vi "rqp_Show FP.vi"(4 "Show in Debugger?":bool=TRUE, 6 "Message Priority":T1=enum."Normal", 7 "Caller in":refnum<class "Worker.lvclass">, 8 "error in":errorcluster, 9 "Data in":T2, 11 "Settings in":refnum<class "Settings.lvclass">) -> (0 "error out":errorcluster, 3 "dup Settings out":refnum<class "Settings.lvclass">, 5 "dup Caller out":refnum<class "Worker.lvclass">)   [LabVIEW 2017, in "Settings.lvclass"]
doc: "This VI sends a <b>Public API Request</b> message to an MHL case of the Worker that owns this VI.\n---\nShow the Front Panel of the Settings Worker's Main VI."
uses:
  Settings.lvclass
  C:/Program Files (x86)/National Instruments/LabVIEW 2017/vi.lib/addons/_Workers/Library/Classes/Worker/Worker.lvclass
  <vilib>/addons/_Workers/Library/Classes/Worker/Worker.lvclass
  rqp_Show FP.ctl
  <vilib>/addons/_Workers/Library/Classes/Message/Priority.ctl
  <vilib>/addons/_Workers/Library/Classes/Worker/Worker.lvclass/Worker.ctl
  <vilib>/addons/_Workers/Library/Classes/Message/Message.lvclass
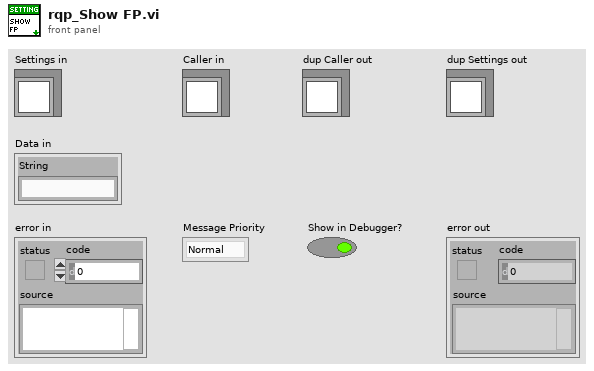
[diagram p1: front panel]
types:
  T1 = typedef "Workers.lvlib/Message.lvclass/Priority.ctl" = enum16{"Low", "Normal", "High"}
  T2 = typedef "Settings.lvclass/rqp_Show FP.ctl" = cluster{"String":string}
  T3 = typedef "Workers.lvlib/Case Label.ctl" = string
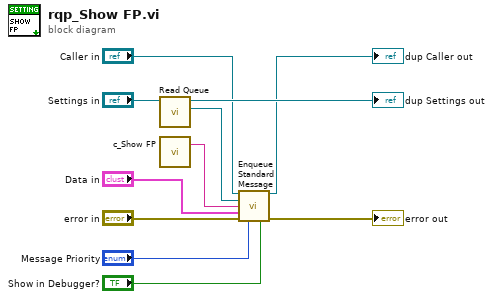
[diagram p0: block diagram]
diagram:
  n1 = call <vilib>:"Read Queue.vi"("Worker_"="Settings in") -> ("Message Queue out"=w5:refnum<class "Message Queue.lvclass">, "dup Worker_out"=→"dup Settings out":refnum<class "Settings.lvclass">)  [unwired: 9 in]
  n2 = call "c_Show FP.vi"() -> ("Case Label"=w4:T3)  [unwired: 1 in]
  n3 = call-dynamic "Enqueue Standard Message.vi"("Worker"="Caller in", "Message Queue"=w5, "Case Label"=w4, "Data"="Data in", "error in (no error)"="error in", "Priority (Normal)"="Message Priority", "Send Message to Debugger? (T)"="Show in Debugger?") -> ("dup Worker out"=→"dup Caller out":refnum<class "Worker.lvclass">, "error out"=→"error out":errorcluster)  [unwired: 7 in]
